vi "Core Actor - INIT - External Queues_Notifiers.vi"(8 "error in (no error)":errorcluster, 11 "Child_2_Class in":refnum<class "SW_Interface_Class.lvclass">) -> (0 "error out":errorcluster, 3 "Child_2_Class out":refnum<class "SW_Interface_Class.lvclass">)   [LabVIEW 2023, in "SW_Interface_Actor.lvlib" / "SW_Interface_Class.lvclass"]
uses:
  SW_Interface_Class.lvclass
  SW_Interface_Class.lvclass/SW_Interface_Class.ctl
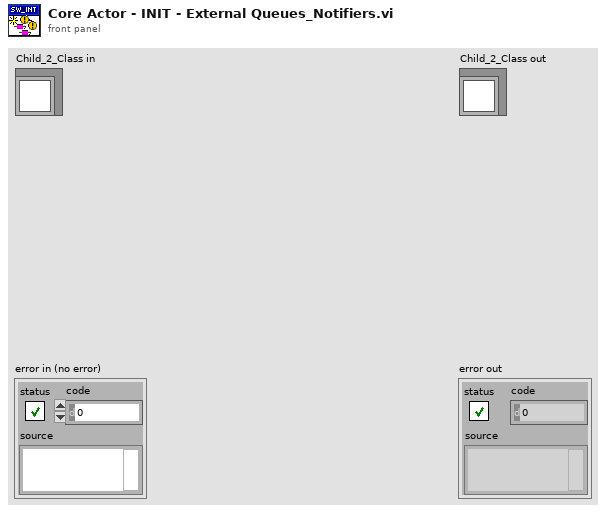
[diagram p1: front panel]
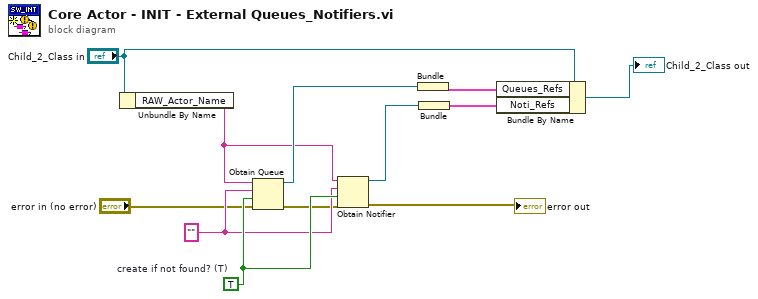
[diagram p0: block diagram]
diagram:
  w8 = TRUE  # create if not found? (T)
  w7 = ""
  n1 = Unbundle By Name("Child_2_Class in") -> ("RAW_Actor_Name"=w2:string)
  n2 = Obtain Queue(name (unnamed)=w2, element data type=w7, create if not found? (T)=w8, error in (no error)="error in (no error)") -> (queue out=w4:refnum<queue>, error out=w6:errorcluster)  [unwired: 1 in, 1 out]
  n3 = Obtain Notifier(name (unnamed)=w2, notification data type=w7, create if not found? (T)=w8, error in (no error)=w6) -> (notifier out=w3:refnum<notifier>, error out=→"error out":errorcluster)  [unwired: 1 out]
  n4 = Bundle("queue out"=w4) -> (w12:cluster{"queue out":refnum<queue>})  [unwired: 1 in]
  n5 = Bundle("notifier out"=w3) -> (w11:cluster{"notifier out":refnum<notifier>})  [unwired: 1 in]
  n6 = Bundle By Name(cluster="Child_2_Class in", "Queues_Refs"=w12, "Noti_Refs"=w11) -> (→"Child_2_Class out":refnum<class "SW_Interface_Class.lvclass">)
